vi "Predict GB via Paralleogram.vi"(10 "Tolerance":dbl=0.001, 11 "Grain Boundary Macro Definition":T2={"Grain 1 Orientation"=[1.0, 0.6019417241891012, 0.029651947654046266], "Grain 2 Orientation"=[1.0, 0.730727623275494, 0.2205637301176], "Twist Angle (Deg)"=0.0}) -> (2 "Grain 2 Monoclinic size":T1={"Height"=1.0, "Width"=1.0, "Angle (deg)"=1.0, "Length"=1.0, "Start"=0.0}, 3 "Grain 1 Monoclinic size":T1={"Height"=1.0, "Width"=1.0, "Angle (deg)"=1.0, "Length"=1.0, "Start"=0.0})   [LabVIEW 2010]
panel:
  out "Grain 2 B":dbl
  out "Grain 1B":dbl
  out "Try this width 2":dbl
  out "A Error 2":dbl
  out "Grain 1 A":dbl
  out "Grain 2 A":dbl
  out "New B2":dbl
  out "New A2":dbl
  out "New C2":dbl
  out "a'":dbl
  out "a1":dbl
  out "Grain 1 C":dbl
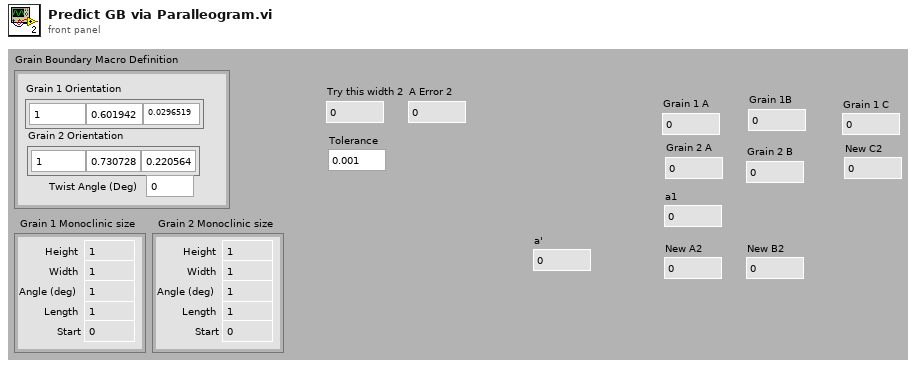
[diagram p1: front panel]
types:
  T1 = cluster{"Height":dbl, "Width":dbl, "Angle (deg)":dbl, "Length":dbl, "Start":dbl}
  T2 = cluster{"Grain 1 Orientation":dbl[], "Grain 2 Orientation":dbl[], "Twist Angle (Deg)":dbl}
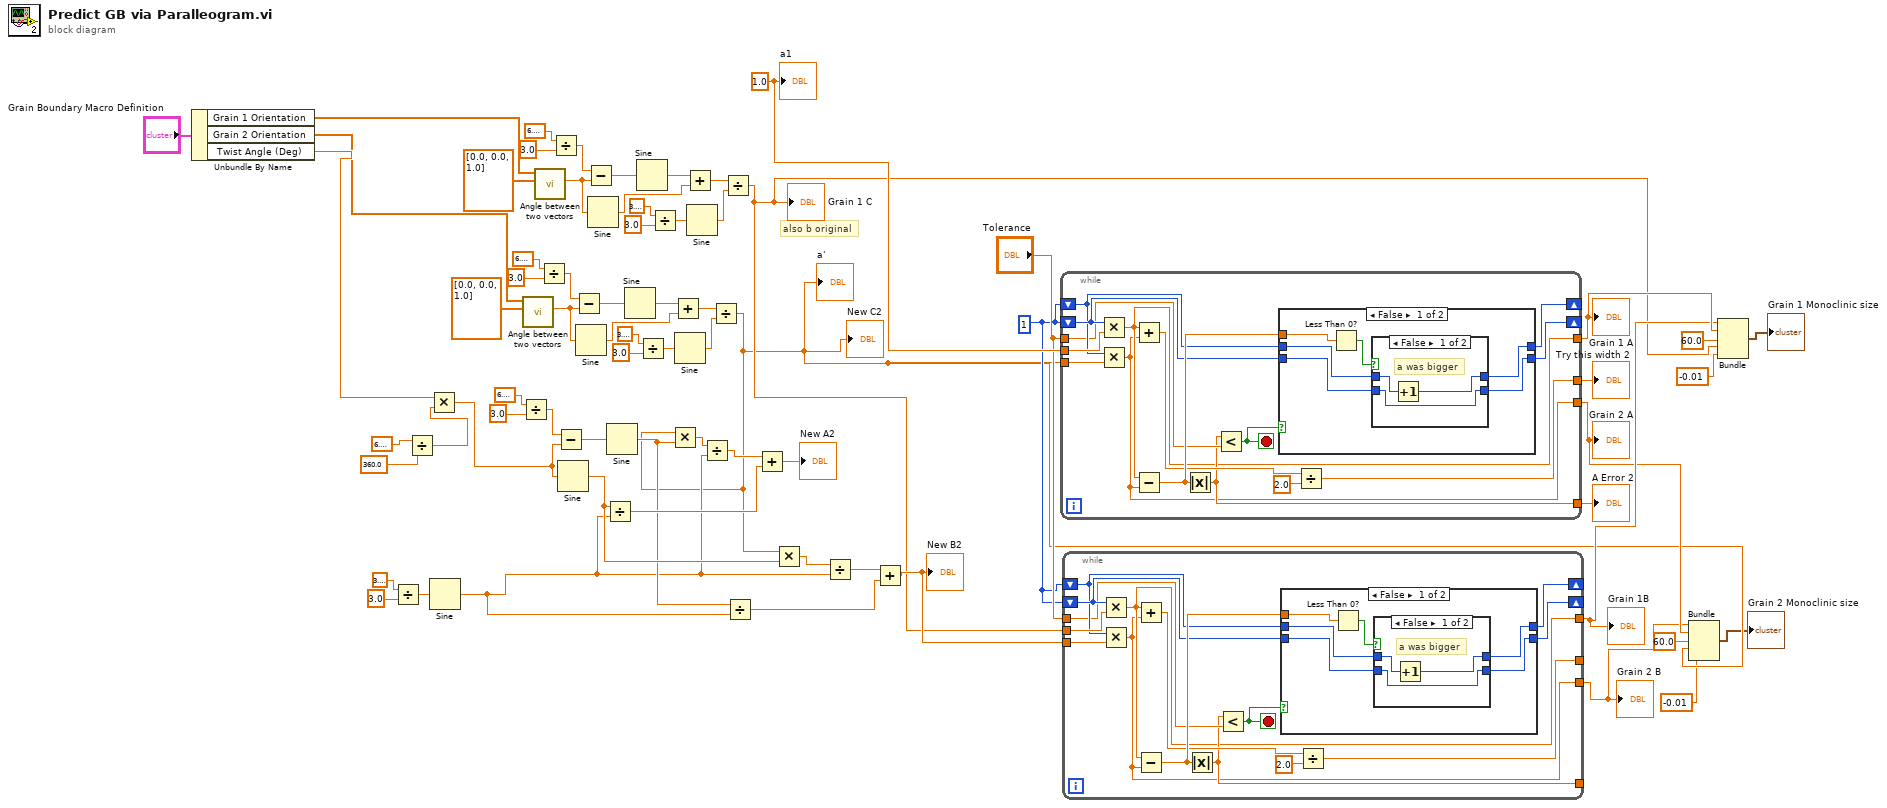
[diagram p0: block diagram]
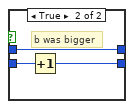
[diagram p2: hidden frame]
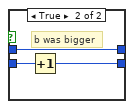
[diagram p4: hidden frame]
diagram:
  w13 = 1
  w16 = 1.0 ("a1")
  # "also b original"
  n1 = Unbundle By Name("Grain Boundary Macro Definition") -> ("Grain 1 Orientation"=w67:dbl[], "Grain 2 Orientation"=w66:dbl[], "Twist Angle (Deg)"=w69:dbl)
  n2 = Divide(x=3.141592653589793, y=3.0) -> (x/y=w37:dbl)
  n3 = Divide(x=6.283185307179586, y=360.0) -> (x/y=w32:dbl)
  n4 = Multiply(x=w69, y=w32) -> (x*y=w33:dbl)
  n5 = Sine(x=w37) -> (sin(x)=w20:dbl)
  n6 = Divide(x=6.283185307179586, y=3.0) -> (x/y=w35:dbl)
  n7 = call "Angle between two vectors.vi"("Vector 2"=dbl[] [0.0, 0.0, 1.0], "Vector 1"=w66) -> ("Angle (Radians)"=w48:dbl)  [unwired: 7 in, 2 out]
  n8 = call "Angle between two vectors.vi"("Vector 2"=dbl[] [0.0, 0.0, 1.0], "Vector 1"=w67) -> ("Angle (Radians)"=w57:dbl)  [unwired: 7 in, 2 out]
  n9 = Divide(x=6.283185307179586, y=3.0) -> (x/y=w46:dbl)
  n10 = Divide(x=6.283185307179586, y=3.0) -> (x/y=w59:dbl)
  n11 = Subtract(x=w35, y=w33) -> (x-y=w34:dbl)
  n12 = Sine(x=w33) -> (sin(x)=w24:dbl)
  n13 = Subtract(x=w46, y=w48) -> (x-y=w47:dbl)
  n14 = Sine(x=w48) -> (sin(x)=w50:dbl)
  n15 = Subtract(x=w59, y=w57) -> (x-y=w58:dbl)
  n16 = Sine(x=w57) -> (sin(x)=w55:dbl)
  n17 = Divide(x=w24, y=w20) -> (x/y=w26:dbl)
  n18 = Sine(x=w34) -> (sin(x)=w21:dbl)
  n19 = Sine(x=w47) -> (sin(x)=w49:dbl)
  n20 = Sine(x=w58) -> (sin(x)=w56:dbl)
  n21 = Divide(x=3.141592653589793, y=3.0) -> (x/y=w42:dbl)
  n22 = Divide(x=3.141592653589793, y=3.0) -> (x/y=w63:dbl)
  n23 = Add(x=w49, y=w50) -> (x+y=w51:dbl)
  n24 = Sine(x=w42) -> (sin(x)=w52:dbl)
  n25 = Add(x=w56, y=w55) -> (x+y=w54:dbl)
  n26 = Sine(x=w63) -> (sin(x)=w53:dbl)
  n27 = Divide(x=w51, y=w52) -> (x/y=w3:dbl)
  "a'" <- w3
  "New C2" <- w3
  n28 = Multiply(x=w3, y=w21) -> (x*y=w28:dbl)
  n29 = Divide(x=w28, y=w20) -> (x/y=w27:dbl)
  n30 = Divide(x=w54, y=w53) -> (x/y=w8:dbl)
  "Grain 1 C" <- w8
  n31 = Divide(x=w21, y=w20) -> (x/y=w19:dbl)
  n32 = Add(x=w27, y=w26) -> (x+y=→"New A2":dbl)
  n33 = Multiply(x=w3, y=w24) -> (x*y=w23:dbl)
  n34 = Divide(x=w23, y=w20) -> (x/y=w22:dbl)
  n35 = Add(x=w22, y=w19) -> (x+y=w14:dbl)
  "New B2" <- w14
  n36 = while {
    shift-right: [w79] -> _
    shift-left: w13 -> [w80]
    shift-right: [w77] -> _
    shift-left: w13 -> [w78]
    tunnel: w16 -> [w84]
    tunnel: w3 -> [w83]
    tunnel: [w73] -> w18
    tunnel: "Tolerance" -> [w76]
    tunnel: [w72] -> w17
    tunnel: [w71] -> w10
    tunnel: [w70] -> w5
    stop <- w82 stop-if-true
    n37 = Multiply(x=w80, y=w84) -> (x*y=w71:dbl)
    n38 = Multiply(x=w78, y=w83) -> (x*y=w70:dbl)
    n39 = Add(x=w71, y=w70) -> (x+y=w74:dbl)
    n40 = Subtract(x=w71, y=w70) -> (x-y=w81:dbl)
    n41 = Absolute Value(x=w81) -> (abs(x)=w72:dbl)
    n42 = Less?(x=w72, y=w76) -> (x < y?=w82:bool)
    n43 = case shown="False" w82 {
      tunnel: w81 -> [w90 _]
      tunnel: w80 -> [w89 w98]
      tunnel: [w88 w98] -> w79
      tunnel: w78 -> [w87 w97]
      tunnel: [w86 w97] -> w77
      frame False {
        n44 = Less Than 0?(x=w90) -> (x < 0?=w85:bool)
        n45 = case shown="False" w85 {
          tunnel: w89 -> [w91 w96]
          tunnel: [w91 w95] -> w88
          tunnel: w87 -> [w93 w94]
          tunnel: [w92 w94] -> w86
          frame False {
            # "a was bigger"
            n46 = Increment(x=w93) -> (x+1=w92:i32)
          }
          frame True {
            # "b was bigger"
            n47 = Increment(x=w96) -> (x+1=w95:i32)
          }
        }
      }
      frame True {
        # "Done"
      }
    }
    n48 = Divide(x=w74, y=2.0) -> (x/y=w73:dbl)
  }
  "Try this width 2" <- w18
  "A Error 2" <- w17
  "Grain 1 A" <- w10
  "Grain 2 A" <- w5
  n49 = while {
    shift-right: [w108] -> _
    shift-left: w13 -> [w109]
    shift-right: [w106] -> _
    shift-left: w13 -> [w107]
    tunnel: w8 -> [w113]
    tunnel: w14 -> [w112]
    tunnel: [w102] -> _
    tunnel: "Tolerance" -> [w105]
    tunnel: [w101] -> _
    tunnel: [w100] -> w9
    tunnel: [w99] -> w4
    stop <- w111 stop-if-true
    n50 = Multiply(x=w109, y=w113) -> (x*y=w100:dbl)
    n51 = Multiply(x=w107, y=w112) -> (x*y=w99:dbl)
    n52 = Add(x=w100, y=w99) -> (x+y=w103:dbl)
    n53 = Subtract(x=w100, y=w99) -> (x-y=w110:dbl)
    n54 = Absolute Value(x=w110) -> (abs(x)=w101:dbl)
    n55 = Less?(x=w101, y=w105) -> (x < y?=w111:bool)
    n56 = case shown="False" w111 {
      tunnel: w110 -> [w119 _]
      tunnel: w109 -> [w118 w127]
      tunnel: [w117 w127] -> w108
      tunnel: w107 -> [w116 w126]
      tunnel: [w115 w126] -> w106
      frame False {
        n57 = Less Than 0?(x=w119) -> (x < 0?=w114:bool)
        n58 = case shown="False" w114 {
          tunnel: w118 -> [w120 w125]
          tunnel: [w120 w124] -> w117
          tunnel: w116 -> [w122 w123]
          tunnel: [w121 w123] -> w115
          frame False {
            # "a was bigger"
            n59 = Increment(x=w122) -> (x+1=w121:i32)
          }
          frame True {
            # "b was bigger"
            n60 = Increment(x=w125) -> (x+1=w124:i32)
          }
        }
      }
      frame True {
        # "Done"
      }
    }
    n61 = Divide(x=w103, y=2.0) -> (x/y=w102:dbl)
  }
  "Grain 1B" <- w9
  "Grain 2 B" <- w4
  n62 = Bundle(w4, w5, "y"=60.0, w3, "y"=-0.01) -> (→"Grain 2 Monoclinic size":cluster{dbl, dbl, "y":dbl, dbl, "y":dbl})  [unwired: 1 in]
  n63 = Bundle(w9, w10, "y"=60.0, w8, "y"=-0.01) -> (→"Grain 1 Monoclinic size":cluster{dbl, dbl, "y":dbl, dbl, "y":dbl})  [unwired: 1 in]
  "a1" <- w16
